vi "3_Mostrar_Señal_del_Generador.vi"() -> ()   [LabVIEW 2020]
panel:
  in  "number of samples":i32=100
  in  "timeout (s)":dbl=10.0 format="%0.2f"
  out "Numeric":dbl
  out "Waveform Chart":dynamicdata(graph)
  in  "milliseconds to wait":u32
  in  "stop":bool
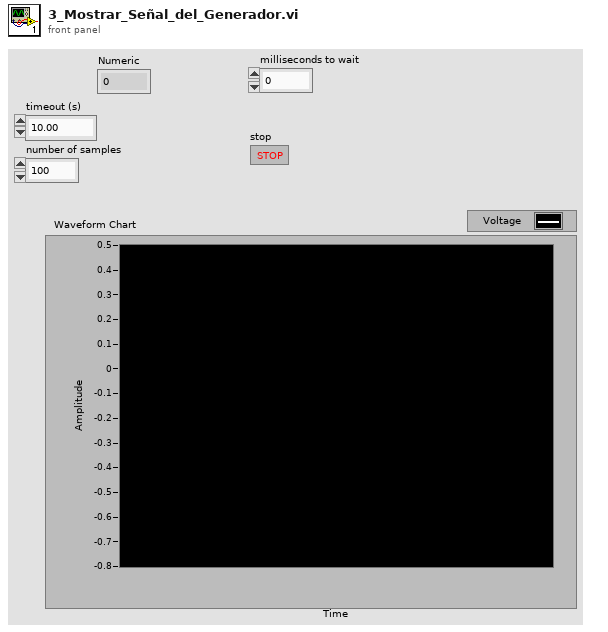
[diagram p1: front panel]
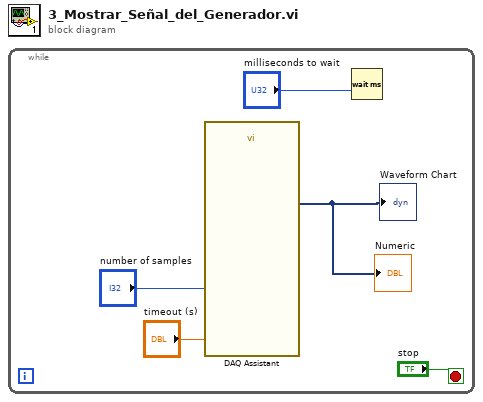
[diagram p0: block diagram]
diagram:
  n1 = while {
    stop <- "stop" stop-if-true
    n2 = call "DAQ Assistant"("number of samples"="number of samples", "timeout (s)"="timeout (s)") -> ("data"=→"Waveform Chart" →"Numeric":dynamicdata)  [unwired: 15 in, 2 out]
    n3 = Wait (ms)(milliseconds to wait="milliseconds to wait") -> ()  [unwired: 1 out]
  }
